vi "serialreadfpga2.vi"(2 "error in":errorcluster caption="error out", 7 "Number of Elements":u32=16, 9 "FPGA VI Reference In":refnum<k20>) -> (0 "Port5":string, 1 "Port8":string, 4 "FPGA VI Reference Out":refnum<k20>, 5 "Port6":string, 6 "Port1":string, 10 "Port2":string, 11 "Port4":string, 12 "Port7":string, 14 "Port3":string, 15 "error out":errorcluster)   [LabVIEW 2010]
uses:
  <vilib>/rvi/interface/nirviMethod/nirviMethod.xnode
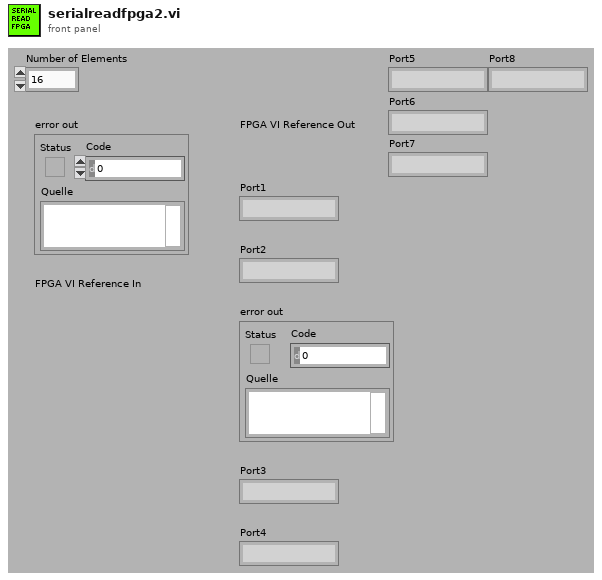
[diagram p1: front panel]
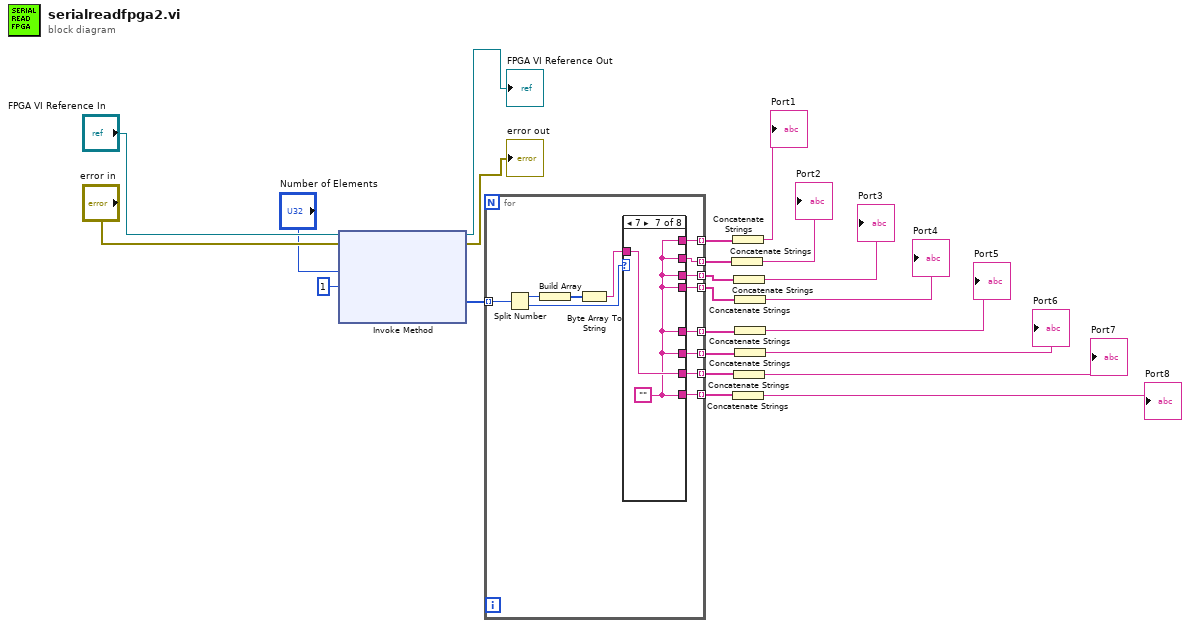
[diagram p0: block diagram]
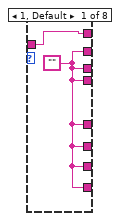
[diagram p2: hidden frame]
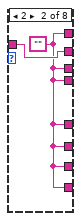
[diagram p3: hidden frame]
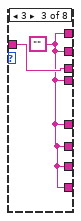
[diagram p4: hidden frame]
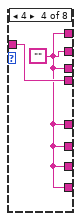
[diagram p5: hidden frame]
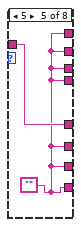
[diagram p6: hidden frame]
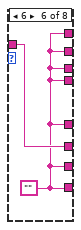
[diagram p7: hidden frame]
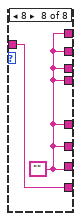
[diagram p8: hidden frame]
diagram:
  n1 = xnode "Invoke Method"("FPGA VI Reference In"="FPGA VI Reference In", "error in"="error in", "Number of Elements"="Number of Elements", "Timeout (ms)"=1) -> ("FPGA VI Reference Out"=→"FPGA VI Reference Out":refnum<k20>, "error out"=→"error out":errorcluster, "Data"=w13:u16[])  [unwired: 1 out]
  n2 = for {
    tunnel: w13 -> [w36] mode=indexing
    tunnel: [w31] -> w18 mode=indexing
    tunnel: [w30] -> w19 mode=indexing
    tunnel: [w29] -> w17 mode=indexing
    tunnel: [w28] -> w16 mode=indexing
    tunnel: [w27] -> w12 mode=indexing
    tunnel: [w26] -> w11 mode=indexing
    tunnel: [w25] -> w10 mode=indexing
    tunnel: [w24] -> w9 mode=indexing
    n3 = Split Number(x=w36) -> (hi(x)=w35:u8, lo(x)=w33:u8)
    n4 = Build Array(w35) -> (w34:u8[])
    n5 = Byte Array To String(unsigned byte array=w34) -> (string=w32:string)
    n6 = case shown="7" w33 {
      tunnel: w32 -> [w38 w40 w42 w44 w46 w48 w50 w52]
      tunnel: [w38 w39 w41 w43 w45 w47 w49 w51] -> w28
      tunnel: [w37 w39 w42 w43 w45 w47 w49 w51] -> w31
      tunnel: [w37 w39 w41 w44 w45 w47 w49 w51] -> w30
      tunnel: [w37 w40 w41 w43 w45 w47 w49 w51] -> w29
      tunnel: [w37 w39 w41 w43 w46 w47 w49 w51] -> w27
      tunnel: [w37 w39 w41 w43 w45 w48 w49 w51] -> w26
      tunnel: [w37 w39 w41 w43 w45 w47 w50 w51] -> w25
      tunnel: [w37 w39 w41 w43 w45 w47 w49 w52] -> w24
      frame 1, Default {
        w37 = ""
      }
      frame 2 {
        w39 = ""
      }
      frame 3 {
        w41 = ""
      }
      frame 4 {
        w43 = ""
      }
      frame 5 {
        w45 = ""
      }
      frame 6 {
        w47 = ""
      }
      frame 7 {
        w49 = ""
      }
      frame 8 {
        w51 = ""
      }
    }
  }
  n7 = Concatenate Strings(w17) -> (→"Port2":string)
  n8 = Concatenate Strings(w16) -> (→"Port1":string)
  n9 = Concatenate Strings(w9) -> (→"Port8":string)
  n10 = Concatenate Strings(w18) -> (→"Port3":string)
  n11 = Concatenate Strings(w10) -> (→"Port7":string)
  n12 = Concatenate Strings(w19) -> (→"Port4":string)
  n13 = Concatenate Strings(w12) -> (→"Port5":string)
  n14 = Concatenate Strings(w11) -> (→"Port6":string)
